vi "Run Tests.vi"   [LabVIEW 2017]
uses:
  <vilib>/addons/_JKI Toolkits/Caraya/run-tests/Run Test (Scalar Path).vi
  <vilib>/addons/_JKI Toolkits/Caraya/Caraya.lvlib
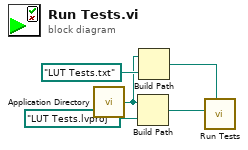
[diagram p0: block diagram]
diagram:
  n1 = call <vilib>:"Application Directory.vi"() -> ("Application Directory"=w3:path)
  n2 = Build Path(base path=w3, name or relative path=path "LUT Tests.lvproj" ("Test Path")) -> (appended path=w1:path)
  n3 = Build Path(base path=w3, name or relative path=path "LUT Tests.txt" ("Test Path")) -> (appended path=w2:path)
  n4 = call-poly <vilib>:"Run Tests.vi"("Report Path"=w2, "Test Path"=w1) -> ()  [unwired: 9 in, 1 out]
